vi "WASH simulation interface.vi"   [LabVIEW 2015]
doc: "Simulates single wash session."
uses:
  type defs/WASH communication module tasks.ctl
  type defs/WASh error handler tasks.ctl
  type defs/WASH simulated database tasks.ctl
types:
  T1 = typedef "WASh error handler tasks.ctl" = enum16{"init", "set current step", "handle error", "close"}
  T2 = typedef "WASH simulated database tasks.ctl" = enum16{"init", "read", "insert record", "update record", "query timing", "close"}
  T3 = typedef "WASH communication module tasks.ctl" = enum16{"init", "enable controls", "update wash indicators", "update wash entry", "update vehicle out of pos", "update timing", "set step buttons values", "set start button value", "set vehicle position entry", "wait for input", "close"}
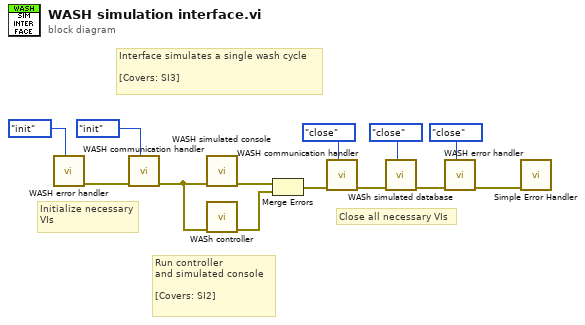
[diagram p0: block diagram]
diagram:
  # "Close all necessary VIs"
  # "Run controller\nand simulated console\n\n[Covers: SI2]"
  # "Initialize necessary\nVIs"
  # "Interface simulates a single wash cycle\n\n[Covers: SI3]"
  n1 = call "WASH error handler.vi"("task"=WASh_error_handler_tasks."init") -> ("error out"=w12:errorcluster)  [unwired: 8 in, 2 out]
  n2 = call "WASH communication handler.vi"("task"=WASH_communication_module_tasks."init", "error in (no error)"=w12) -> ("error out"=w13:errorcluster)  [unwired: 6 in, 3 out]
  n3 = call "WASH simulated console.vi"("error in (no error)"=w13) -> ("error out"=w9:errorcluster)  [unwired: 10 in]
  n4 = call "WASh controller.vi"("error in (no error)"=w13) -> ("error out"=w8:errorcluster)  [unwired: 10 in]
  n5 = Merge Errors(w9, w8) -> (w7:errorcluster)
  n6 = call "WASH communication handler.vi"("task"=WASH_communication_module_tasks."close", "error in (no error)"=w7) -> ("error out"=w5:errorcluster)  [unwired: 6 in, 3 out]
  n7 = call "WASh simulated database.vi"("task"=WASH_simulated_database_tasks."close", "error in (no error)"=w5) -> ("error out"=w2:errorcluster)  [unwired: 7 in, 2 out]
  n8 = call "WASH error handler.vi"("task"=WASh_error_handler_tasks."close", "error in (no error)"=w2) -> ("error out"=w1:errorcluster)  [unwired: 7 in, 2 out]
  n9 = call <vilib>:"Simple Error Handler.vi"("error in (no error)"=w1) -> ()  [unwired: 4 in, 5 out]
